vi "get graphs from spots.vi"(7 "n points in graph":dbl=0.2, 8 "pos history time":dbl=10.0, 9 "photon history time":dbl=60.0, 10 "photon graph type":enum16{"red", "green", "ratio"}(ring), 11 "spots":T2(array[cluster])) -> (1 "spot locations":T1[](array[typedef]), 2 "position graphs":cluster{"yi":dbl[], "yi":dbl[]}[](array[cluster]), 3 "photon graphs":cluster{"t values":dbl[], "x values":dbl[]}[](array[cluster]))   [LabVIEW 2010]
uses:
  spot location.ctl
  <vilib>/Analysis/1siggen.llb/Ramp Pattern by Delta.vi
  <vilib>/gmath/NI_Gmath.lvlib
  <vilib>/Analysis/NI_AALBase.lvlib
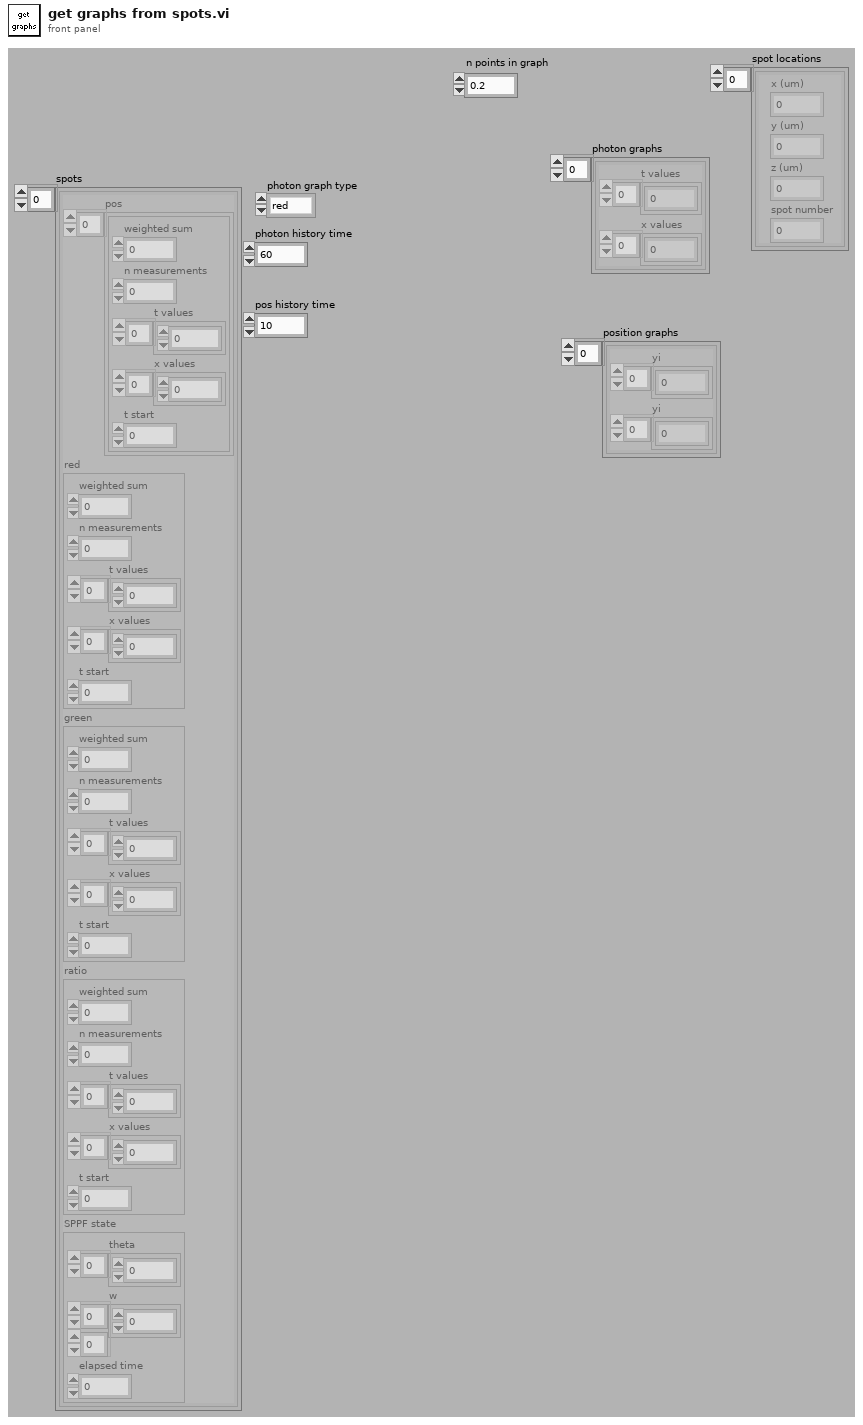
[diagram p1: front panel]
types:
  T1 = typedef "spot location.ctl" = cluster{"x (um)":dbl, "y (um)":dbl, "z (um)":dbl, "spot number":u8}
  T2 = cluster{"pos":cluster{"weighted sum":dbl, "n measurements":dbl, "t values":dbl[], "x values":dbl[], "t start":dbl}[], "red":cluster{"weighted sum":dbl, "n measurements":dbl, "t values":dbl[], "x values":dbl[], "t start":dbl}, "green":cluster{"weighted sum":dbl, "n measurements":dbl, "t values":dbl[], "x values":dbl[], "t start":dbl}, "ratio":cluster{"weighted sum":dbl, "n measurements":dbl, "t values":dbl[], "x values":dbl[], "t start":dbl}, "SPPF state":cluster{"theta":dbl[], "w":dbl[][], "elapsed time":dbl}}[]
  T3 = cluster{"weighted sum":dbl, "n measurements":dbl, "t values":dbl[], "x values":dbl[], "t start":dbl}
  T4 = cluster{"weighted sum":dbl, "n measurements":dbl, "t values":dbl[], "x values":dbl[], "t start":dbl}[]
  T5 = cluster{"pos[0]":cluster{"weighted sum":dbl, "n measurements":dbl, "t values":dbl[], "x values":dbl[], "t start":dbl}, "pos[1]":cluster{"weighted sum":dbl, "n measurements":dbl, "t values":dbl[], "x values":dbl[], "t start":dbl}, "pos[2]":cluster{"weighted sum":dbl, "n measurements":dbl, "t values":dbl[], "x values":dbl[], "t start":dbl}}
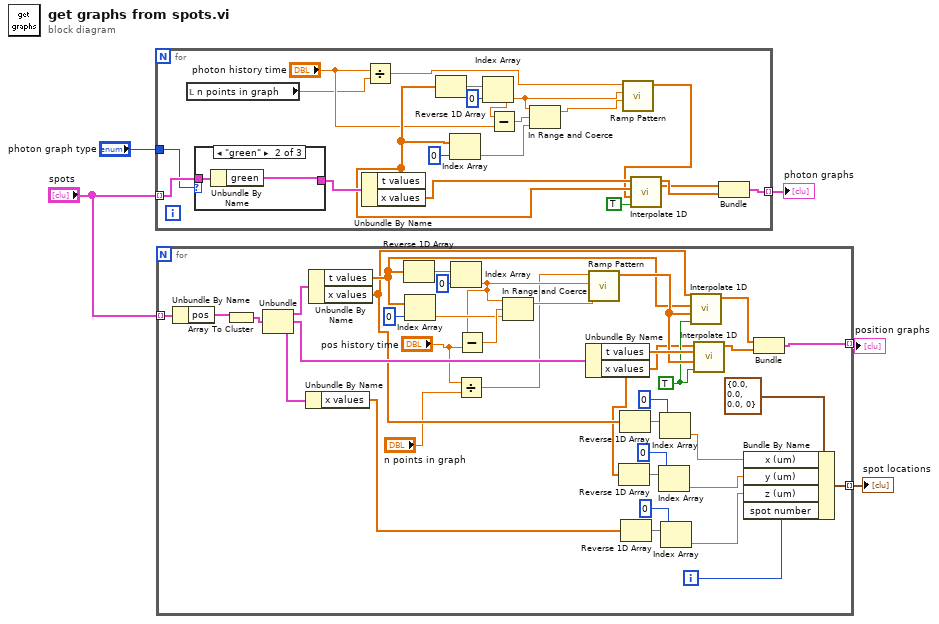
[diagram p0: block diagram]
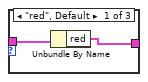
[diagram p2: hidden frame]
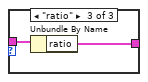
[diagram p3: hidden frame]
diagram:
  n1 = for {
    tunnel: "spots" -> [w25] mode=indexing
    tunnel: [w23] -> w4 mode=indexing
    tunnel: "photon graph type" -> [w22]
    n2 = local read "n points in graph"() -> (w7:dbl)
    n3 = case shown="\"green\"" w22 {
      tunnel: w25 -> [w27 w29 w31]
      tunnel: [w26 w28 w30] -> w24
      frame "red", Default {
        n4 = Unbundle By Name(w27) -> ("red"=w26:T3)
      }
      frame "green" {
        n5 = Unbundle By Name(w29) -> ("green"=w28:T3)
      }
      frame "ratio" {
        n6 = Unbundle By Name(w31) -> ("ratio"=w30:T3)
      }
    }
    n7 = Unbundle By Name(w24) -> ("t values"=w14:dbl[], "x values"=w13:dbl[])
    n8 = Divide(x="photon history time", y=w7) -> (x/y=w6:dbl)
    n9 = Reverse 1D Array(array=w14) -> (reversed array=w21:dbl[])
    n10 = Index Array(array=w14, index=0) -> (element=w18:dbl)
    n11 = Index Array(array=w21, index=0) -> (element=w16:dbl)
    n12 = Subtract(x=w16, y="photon history time") -> (x-y=w19:dbl)
    n13 = In Range and Coerce(upper limit=w16, x=w19, lower limit=w18) -> (coerced(x)=w15:dbl)  [unwired: 1 out]
    n14 = call-poly <vilib>:"Ramp Pattern.vi"("start"=w15, "end"=w16, "delta"=w6) -> ("Ramp Pattern"=w12:dbl[])  [unwired: 6 in, 2 out]
    n15 = call <vilib>:"Interpolate 1D.vi"("X is monotonic"=TRUE, "xi"=w12, "X"=w14, "Y"=w13) -> ("xi used"=w10:dbl[], "yi"=w11:dbl[])  [unwired: 5 in, 1 out]
    n16 = Bundle("xi used"=w10, "yi"=w11) -> (w23:cluster{"xi used":dbl[], "yi":dbl[]})  [unwired: 1 in]
  }
  "photon graphs" <- w4
  n17 = for {
    tunnel: "spots" -> [w69] mode=indexing
    tunnel: [w58] -> w2 mode=indexing
    tunnel: [w35] -> w1 mode=indexing
    i -> [w36]
    w51 = TRUE ("X is monotonic")
    n18 = Unbundle By Name(w69) -> ("pos"=w68:T4)
    n19 = Array To Cluster(array=w68) -> (cluster=w67:T5)
    n20 = Unbundle(w67) -> ("pos[0]"=w66:T3, "pos[1]"=w63:T3, "pos[2]"=w50:T3)
    n21 = Unbundle By Name(w50) -> ("x values"=w41:dbl[])
    n22 = Unbundle By Name(w66) -> ("t values"=w55:dbl[], "x values"=w43:dbl[])
    n23 = Reverse 1D Array(array=w55) -> (reversed array=w65:dbl[])
    n24 = Index Array(array=w55, index=0) -> (element=w53:dbl)
    n25 = Index Array(array=w65, index=0) -> (element=w52:dbl)
    n26 = Divide(x="pos history time", y="n points in graph") -> (x/y=w32:dbl)
    n27 = Subtract(x=w52, y="pos history time") -> (x-y=w56:dbl)
    n28 = In Range and Coerce(upper limit=w52, x=w56, lower limit=w53) -> (coerced(x)=w57:dbl)  [unwired: 1 out]
    n29 = Unbundle By Name(w63) -> ("t values"=w62:dbl[], "x values"=w42:dbl[])
    n30 = call-poly <vilib>:"Ramp Pattern.vi"("start"=w57, "end"=w52, "delta"=w32) -> ("Ramp Pattern"=w61:dbl[])  [unwired: 6 in, 2 out]
    n31 = Reverse 1D Array(array=w42) -> (reversed array=w47:dbl[])
    n32 = Reverse 1D Array(array=w43) -> (reversed array=w49:dbl[])
    n33 = Reverse 1D Array(array=w41) -> (reversed array=w45:dbl[])
    n34 = Index Array(array=w47, index=0) -> (element=w38:dbl)
    n35 = Index Array(array=w49, index=0) -> (element=w39:dbl)
    n36 = Index Array(array=w45, index=0) -> (element=w37:dbl)
    n37 = call <vilib>:"Interpolate 1D.vi"("X is monotonic"=w51, "xi"=w61, "X"=w55, "Y"=w43) -> ("yi"=w59:dbl[])  [unwired: 5 in, 2 out]
    n38 = call <vilib>:"Interpolate 1D.vi"("X is monotonic"=w51, "xi"=w61, "X"=w62, "Y"=w42) -> ("yi"=w60:dbl[])  [unwired: 5 in, 2 out]
    n39 = Bundle By Name(cluster=T1 {"x (um)"=0.0, "y (um)"=0.0, "z (um)"=0.0, "spot number"=0} ("location"), "x (um)"=w39, "y (um)"=w38, "z (um)"=w37, "spot number"=w36) -> (w35:T1)
    n40 = Bundle("yi"=w59, "yi"=w60) -> (w58:cluster{"yi":dbl[], "yi":dbl[]})  [unwired: 1 in]
  }
  "position graphs" <- w2
  "spot locations" <- w1
